vi "simx Query.vi"(0 "clientID":i32, 1 "retSignalName":string, 2 "retSignalLength":i32, 5 "signalName":string, 7 "signalValue":string, 9 "signalLength":i32, 11 "error in (no error)":errorcluster, 12 "retSignalValue":string, 13 "timeOutInMs":i32) -> (4 "retSignalLength out":i32, 6 "function return":i32, 14 "retSignalValue out":string, 15 "error out":errorcluster)   [LabVIEW 2019, in "PXL_V-REP.lvlib"]
doc: "EXTAPI_DLLEXPORT simxInt simxQuery(simxInt clientID,const simxChar* signalName,const simxUChar* signalValue,simxInt signalLength,const simxChar* retSignalName,simxUChar** retSignalValue,simxInt* retSignalLength,simxInt timeOutInMs);"
uses:
  PXL_V-REP.lvlib
  <userlib>/V-REP/remoteApi.dll
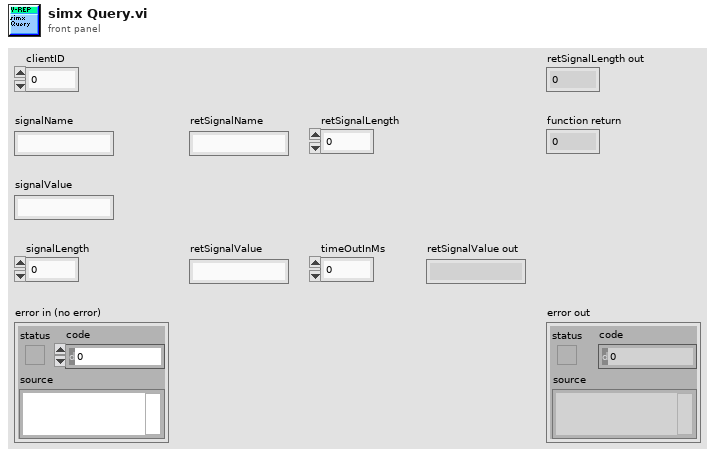
[diagram p1: front panel]
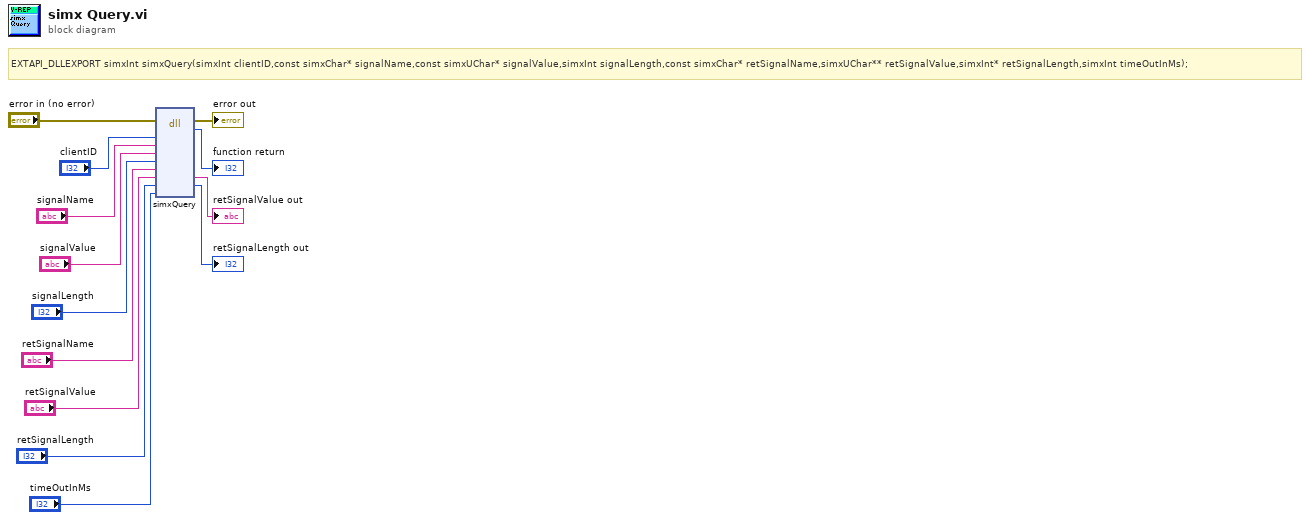
[diagram p0: block diagram]
diagram:
  # "EXTAPI_DLLEXPORT simxInt simxQuery(simxInt clientID,const simxChar* signalName,const simxUChar* signalValue,simxInt signalLength,const simxChar* retSignalName,simxUChar** retSignalValue,simxInt* retSignalLength,simxInt timeOutInMs);"
  n1 = dll-call lib="C:/Program Files (x86)/National Instruments/LabVIEW 2019/user.lib/V-REP/remoteApi.*" fn="simxQuery"(error in="error in (no error)", "clientID"="clientID", "signalName"="signalName", "signalValue"="signalValue", "signalLength"="signalLength", "retSignalName"="retSignalName", "retSignalValue"="retSignalValue", "retSignalLength"="retSignalLength", "timeOutInMs"="timeOutInMs") -> (error out=→"error out":errorcluster, →"function return":i32, "retSignalValue"=→"retSignalValue out":string, "retSignalLength"=→"retSignalLength out":i32)  [unwired: 8 in, 1 out]
